vi "Get_Trace_andUnit (SubVI).vi"(0 "Filter?":bool, 4 "Array":i32[](array[numeric]), 5 "max points per trace (all)":i32=-1, 6 "time interval":T2, 7 "database URL":path=path "\\\\HousesoftheHoly\\Default_Database", 8 "options":T1={"interpolate data (F)"=FALSE, "extrapolate to now (F)"=FALSE, "remove data breaks (F)"=FALSE, "interpolation interval (1 s)"=1.0, "maintain trending info (T)"=TRUE} {"interpolation interval (1 s)" min=0.0 format="%0.2f"}, 9 "Array in":string[](array[string]), 10 "XYGraph Refnum":refnum<vi>, 11 "XYGraph in":refnum<vi>) -> (3 "Array out":T3(array[cluster]))   [LabVIEW 2016]
uses:
  <vilib>/lvdsc/historical/Read Trace (Numeric).vi
  <vilib>/lvdsc/NI_DSC.lvlib
  <vilib>/Analysis/NI_AALBase.lvlib
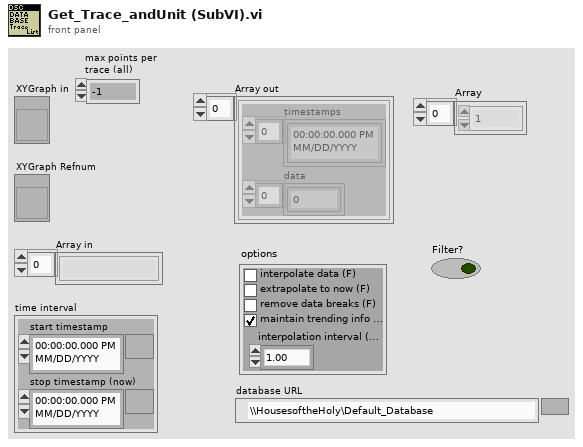
[diagram p1: front panel]
types:
  T1 = cluster{"interpolate data (F)":bool, "extrapolate to now (F)":bool, "remove data breaks (F)":bool, "interpolation interval (1 s)":dbl, "maintain trending info (T)":bool}
  T2 = cluster{"start timestamp":timestamp, "stop timestamp (now)":timestamp}
  T3 = cluster{"timestamps":timestamp[], "data":dbl[]}[]
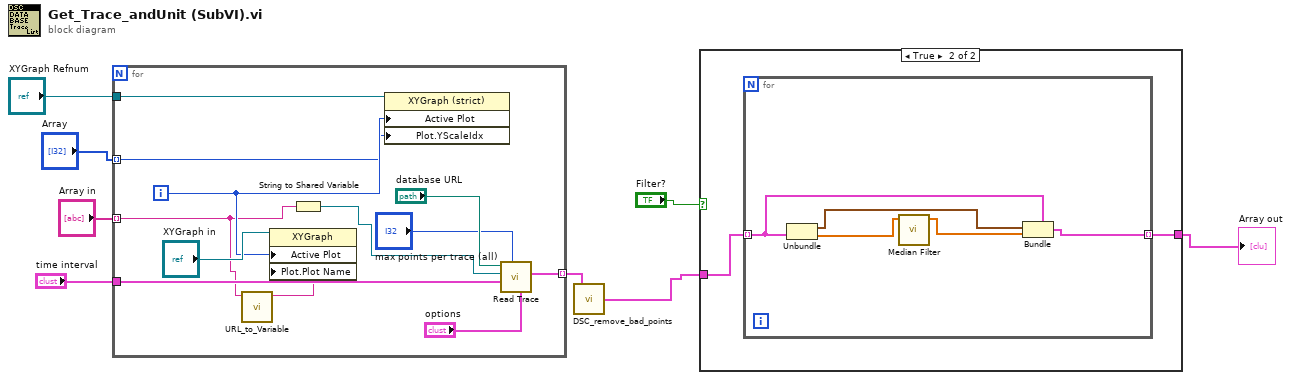
[diagram p0: block diagram]
diagram:
  n1 = for {
    tunnel: "Array in" -> [w10] mode=indexing
    tunnel: [w17] -> w5 mode=indexing
    tunnel: "time interval" -> [w19]
    tunnel: "XYGraph Refnum" -> [w16]
    tunnel: "Array" -> [w13] mode=indexing
    i -> [w15]
    n2 = call "URL_to_Variable.vi"("URL"=w10) -> ("Name"=w9:string)  [unwired: 10 in]
    n3 = property on="Property Node" class="XYGraph"(reference="XYGraph in", "Active Plot"=w15, "Plot.Plot Name"=w9) -> ()  [unwired: 1 in, 2 out]
    n4 = String to Shared Variable(0:w10) -> (2:w11:refnum<k21>)  [unwired: 1 out]
    n5 = property on="Property Node" class="XYGraph (strict)"(reference=w16, "Active Plot"=w15, "Plot.YScaleIdx"=w13) -> ()  [unwired: 1 in, 2 out]
    n6 = call-poly <vilib>:"Read Trace.vi"("options"="options", "max points per trace (all)"="max points per trace (all)", "time interval"=w19, "trace name"=w11, "database URL"="database URL") -> ("historical trace"=w17:cluster{"timestamps":timestamp[], "data":dbl[]})  [unwired: 3 in, 3 out]
  }
  n7 = call "DSC_remove_bad_points.vi"("Database Trace In"=w5) -> ("Database Trace Out"=w3:T3)
  n8 = case shown="True" "Filter?" {
    tunnel: w3 -> [w21 w23]
    tunnel: [w21 w22] -> w1
    frame False {
    }
    frame True {
      n9 = for {
        tunnel: w23 -> [w28] mode=indexing
        tunnel: [w24] -> w22 mode=indexing
        n10 = Unbundle(w28) -> ("timestamps"=w26:timestamp[], "data"=w27:dbl[])
        n11 = call <vilib>:"Median Filter.vi"("X"=w27) -> ("Filtered X"=w25:dbl[])  [unwired: 9 in, 1 out]
        n12 = Bundle(cluster=w28, "timestamps"=w26, "data"=w25) -> (w24:cluster{"timestamps":timestamp[], "data":dbl[]})
      }
    }
  }
  "Array out" <- w1
